vi "oax_Set All Menus.vi"(6 "enabled":bool, 8 "error in (no error)":errorcluster, 11 "menu reference":refnum<k9>) -> (0 "error out":errorcluster)   [LabVIEW 2017]
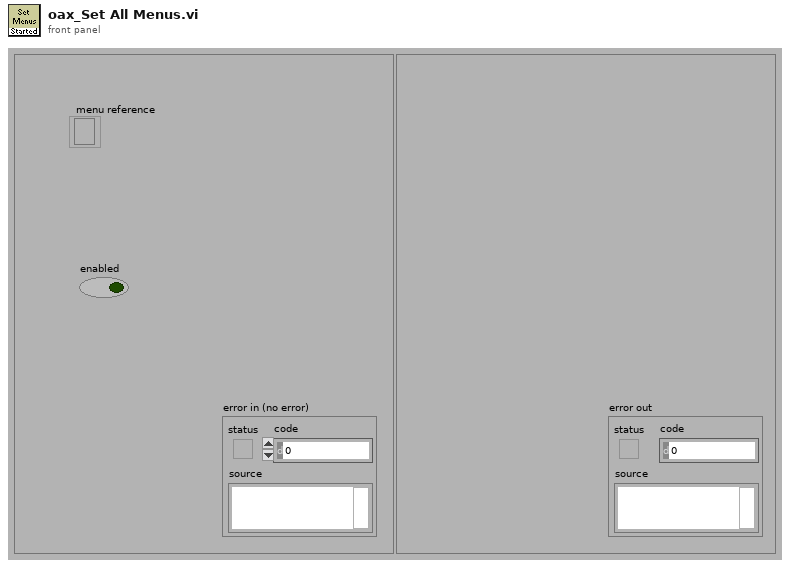
[diagram p1: front panel]
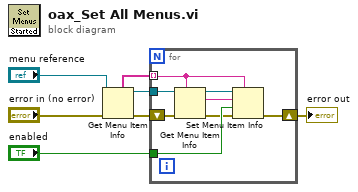
[diagram p0: block diagram]
diagram:
  n1 = Get Menu Item Info(8:"error in (no error)", 11:"menu reference") -> (0:w3:errorcluster, 3:w5:refnum<k9>, 5:w6:string[])  [unwired: 1 in, 4 out]
  n2 = for {
    tunnel: w6 -> [w15] mode=indexing
    tunnel: w5 -> [w13]
    tunnel: "enabled" -> [w11]
    shift-right: [w8] -> w1
    shift-left: w3 -> [w10]
    n3 = Get Menu Item Info(7:w15, 8:w10, 11:w13) -> (0:w9:errorcluster, 2:w14:string, 3:w12:refnum<k9>)  [unwired: 4 out]
    n4 = Set Menu Item Info(7:w15, 8:w9, 9:w11, 10:w14, 11:w12) -> (0:w8:errorcluster)  [unwired: 2 in, 1 out]
  }
  "error out" <- w1
